vi "FindInstrument.vi"(6 "search string/char ()":string, 8 "error in (no error)":errorcluster) -> (0 "error out":errorcluster, 1 "Found Interface Names":string[](array[string]), 2 "Found Resource Names":string[](array[string]))   [LabVIEW 2020, in "FCR100.lvlib"]
doc: "Query the Instruments in the system.\n\nFinds and connects through VISA.\n\nsearch string:\nSearch string can be used to filter results to a particular type that has search string in it Interface Name. It is optional and blank by default.\n\nOutput Found Resource Names are VISA Resource names and Found Interface Names are the matching Interface names."
uses:
  <vilib>/Instr/_visa.llb/VISA Find Search Mode.ctl
  FCR100.lvlib
panel:
  # "Newport Find Instruments"
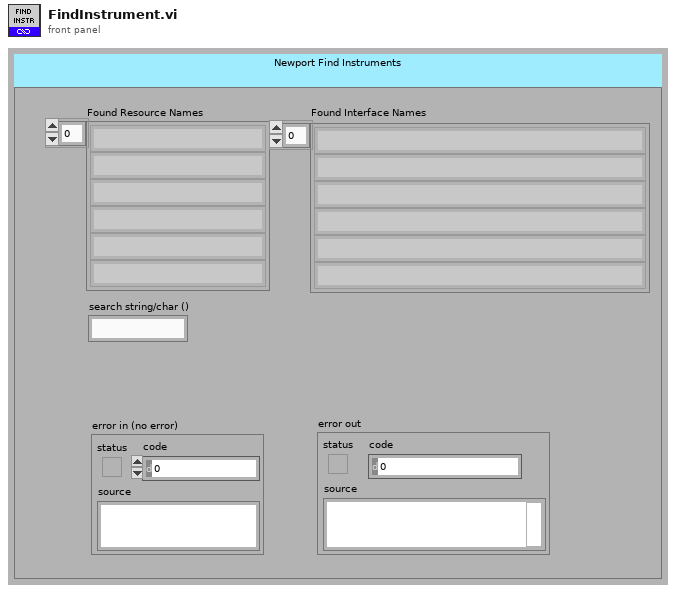
[diagram p1: front panel]
types:
  T1 = typedef "VISA Find Search Mode.ctl" = u32
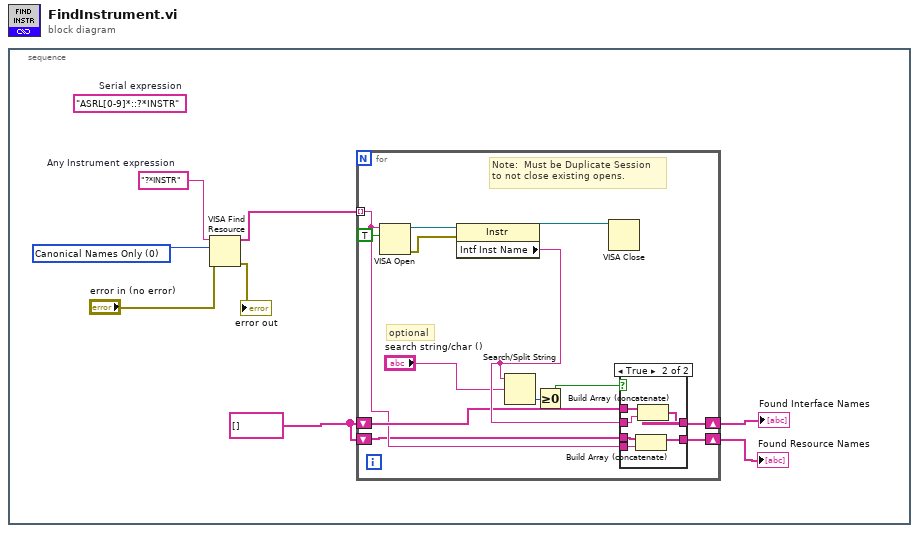
[diagram p0: block diagram]
diagram:
  n1 = stacked-sequence {
    frame #0 {
      (unwired) "ASRL[0-9]*::?*INSTR"  # Serial expression
      w3 = string[] [] ("Array 2")
      w4 = T1 0 items=["Canonical Names Only"=0, "Aliases Only"=2, "Include Matching Aliases"=3, "Include All Aliases"=4] ("Search Mode")
      w5 = "?*INSTR"  # Any Instrument expression
      n2 = VISA Find Resource(8:"error in (no error)", 10:w4, 11:w5) -> (0:→"error out":errorcluster, 3:w7:string[])  [unwired: 1 out]
      n3 = for {
        tunnel: w7 -> [w14] mode=indexing
        shift-right: [w17] -> w6
        shift-left: w3 -> [w15]
        shift-right: [w12] -> w2
        shift-left: w3 -> [w13]
        # "Note:  Must be Duplicate Session\nto not close existing opens."
        # "optional"
        n4 = VISA Open(duplicate session (F)=TRUE, VISA resource name=w14) -> (VISA resource name=w21:refnum<visa-resource-name>, error out=w20:errorcluster)  [unwired: 3 in]
        n5 = property class="Instr"(reference=w21, error in=w20) -> (reference out=w9:refnum<visa-resource-name>, "Intf Inst Name"=w16:string)  [unwired: 1 out]
        n6 = Search/Split String(string=w16, search string/char (-)="search string/char ()") -> (offset of match=w19:i32)  [unwired: 1 in, 2 out]
        n7 = Greater Or Equal To 0?(x=w19) -> (x >= 0?=w18:bool)
        n8 = VISA Close(VISA resource name=w9) -> ()  [unwired: 1 in, 1 out]
        n9 = case shown="True" w18 {
          tunnel: w15 -> [w23 w28]
          tunnel: [w23 w29] -> w17
          tunnel: w16 -> [_ w27]
          tunnel: w14 -> [_ w26]
          tunnel: w13 -> [w22 w25]
          tunnel: [w22 w24] -> w12
          frame False {
          }
          frame True {
            n10 = Build Array (concatenate)(w25, w26) -> (w24:string[])
            n11 = Build Array (concatenate)(w28, w27) -> (w29:string[])
          }
        }
      }
      "Found Resource Names" <- w2
      "Found Interface Names" <- w6
    }
  }
